vi "AddOrder.vi"(11 "buffer.in":u64[](array[numeric])=[2459274161843883858, 5279397646710161952, 5620492615227034656, 281474976710656, 0, 0, 0, 0, 0] format="%.0x") -> (3 "OrderBook.Command":T1={"type"=enum."AddOrder", "side"=66, "orderId "=3544385890602799695, "quantity"=20000, "symbol"=138719281473, "price"=1, "executed.qty"=0, "canceled.qty"=0, "remaining.qty"=0, "seconds"=0, "nanoseconds"=447000, "Add"=FALSE, "Edit"=FALSE, "Remove"=FALSE} {"symbol" format="%.0x"})   [LabVIEW 2020]
uses:
  builds/fpganow.common/orderbook.command.ctl
  builds/fpganow.common/orderbook.command.type.ctl
  Market.Data.Common/fpga/fpganow.common.fpga.lvlib
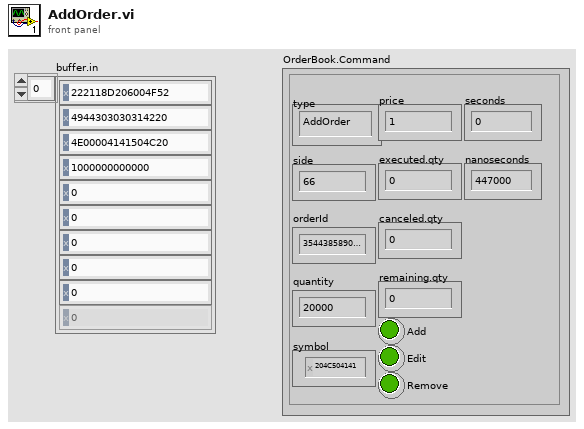
[diagram p1: front panel]
types:
  T1 = typedef "fpganow.common.fpga.lvlib/orderbook.command.ctl" = cluster{"type":T2, "side":u8, "orderId ":u64, "quantity":u32, "symbol":u64, "price":u64, "executed.qty":u32, "canceled.qty":u32, "remaining.qty":u32, "seconds":u64, "nanoseconds":u64, "Add":bool, "Edit":bool, "Remove":bool}
  T2 = typedef "fpganow.common.fpga.lvlib/orderbook.command.type.ctl" = enum8{"Time", "AddOrder", "OrderExecuted", "OrderExecutedAtPrice", "ReduceSize", "ModifyOrder", "DeleteOrder", "Get.Everything", "Get.All.Orders", "Get.Top"}
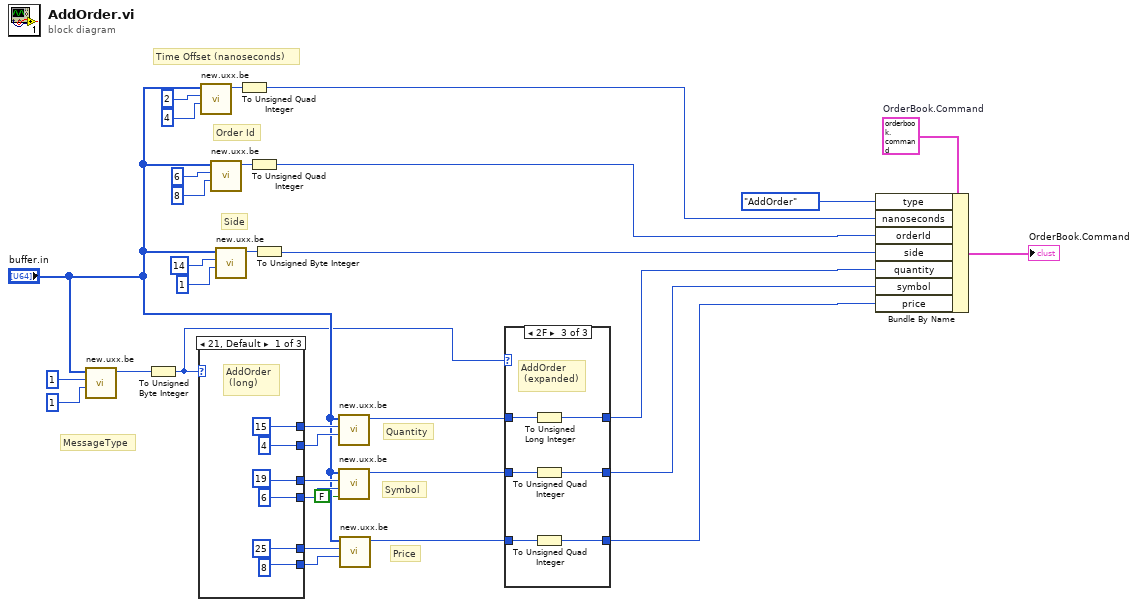
[diagram p0: block diagram]
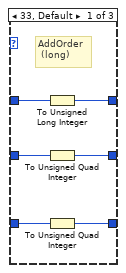
[diagram p2: hidden frame]
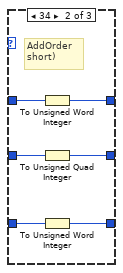
[diagram p3: hidden frame]
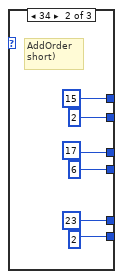
[diagram p4: hidden frame]
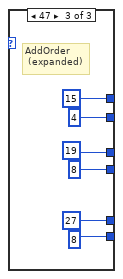
[diagram p5: hidden frame]
diagram:
  w30 = T1 {"type"=enum."AddOrder", "side"=0, "orderId "=0, "quantity"=0, "symbol"=0, "price"=0, "executed.qty"=0, "canceled.qty"=0, "remaining.qty"=0, "seconds"=0, "nanoseconds"=0, "Add"=FALSE, "Edit"=FALSE, "Remove"=FALSE}  # OrderBook.Command
  # "Price"
  # "Symbol"
  # "Quantity"
  # "Side"
  # "Order Id"
  # "Time Offset (nanoseconds)"
  # "MessageType"
  n1 = call "new.uxx.be.vi"("buffer (U64)"="buffer.in", "Start.Idx"=u8 1, "Length"=u8 1) -> ("Uxx.be"=w31:u64)  [unwired: 7 in]
  n2 = To Unsigned Byte Integer(number=w31) -> (unsigned 8bit integer=w5:u8)
  n3 = case shown="21, Default" w5 {
    tunnel: [u8 15 ("Start.Idx") u8 15 ("Start.Idx") u8 15 ("Start.Idx")] -> w12
    tunnel: [u8 4 ("Length") u8 2 ("Length") u8 4 ("Length")] -> w11
    tunnel: [u8 19 ("Start.Idx") u8 17 ("Start.Idx") u8 19 ("Start.Idx")] -> w10
    tunnel: [u8 6 ("Length") u8 6 ("Length") u8 8 ("Length")] -> w9
    tunnel: [u8 25 ("Start.Idx") u8 23 ("Start.Idx") u8 27 ("Start.Idx")] -> w8
    tunnel: [u8 8 ("Length") u8 2 ("Length") u8 8 ("Length")] -> w7
    frame 33, Default {
      # "AddOrder\n (long)"
    }
    frame 34 {
      # "AddOrder \nshort)"
    }
    frame 47 {
      # "AddOrder\n (expanded)"
    }
  }
  n4 = call "new.uxx.be.vi"("buffer (U64)"="buffer.in", "Start.Idx"=u8 2, "Length"=u8 4) -> ("Uxx.be"=w25:u64)  [unwired: 7 in]
  n5 = call "new.uxx.be.vi"("buffer (U64)"="buffer.in", "Start.Idx"=u8 6, "Length"=u8 8) -> ("Uxx.be"=w22:u64)  [unwired: 7 in]
  n6 = call "new.uxx.be.vi"("buffer (U64)"="buffer.in", "Start.Idx"=u8 14, "Length"=u8 1) -> ("Uxx.be"=w19:u64)  [unwired: 7 in]
  n7 = To Unsigned Quad Integer(1:w25) -> (0:w15:u64)
  n8 = To Unsigned Quad Integer(1:w22) -> (0:w14:u64)
  n9 = To Unsigned Byte Integer(number=w19) -> (unsigned 8bit integer=w13:u8)
  n10 = call "new.uxx.be.vi"("buffer (U64)"="buffer.in", "Start.Idx"=w12, "Length"=w11) -> ("Uxx.be"=w18:u64)  [unwired: 7 in]
  n11 = call "new.uxx.be.vi"("buffer (U64)"="buffer.in", "Start.Idx"=w10, "Length"=w9, "Big.Endian?"=FALSE) -> ("Uxx.be"=w17:u64)  [unwired: 6 in]
  n12 = call "new.uxx.be.vi"("buffer (U64)"="buffer.in", "Start.Idx"=w8, "Length"=w7) -> ("Uxx.be"=w16:u64)  [unwired: 7 in]
  n13 = case shown="2F" w5 {
    tunnel: [w54 w60 w66] -> w4
    tunnel: [w53 w59 w65] -> w3
    tunnel: [w52 w58 w64] -> w2
    tunnel: w18 -> [w57 w61 w68]
    tunnel: w16 -> [w55 w63 w69]
    tunnel: w17 -> [w56 w62 w67]
    frame 33, Default {
      # "AddOrder\n (long)"
      n14 = To Unsigned Long Integer(number=w57) -> (unsigned 32bit integer=w54:u32)
      n15 = To Unsigned Quad Integer(1:w56) -> (0:w53:u64)
      n16 = To Unsigned Quad Integer(1:w55) -> (0:w52:u64)
    }
    frame 34 {
      # "AddOrder \nshort)"
      n17 = To Unsigned Word Integer(number=w61) -> (unsigned 16bit integer=w60:u16)
      n18 = To Unsigned Quad Integer(1:w62) -> (0:w59:u64)
      n19 = To Unsigned Word Integer(number=w63) -> (unsigned 16bit integer=w58:u16)
    }
    frame 47 {
      # "AddOrder\n (expanded)"
      n20 = To Unsigned Long Integer(number=w68) -> (unsigned 32bit integer=w66:u32)
      n21 = To Unsigned Quad Integer(1:w67) -> (0:w65:u64)
      n22 = To Unsigned Quad Integer(1:w69) -> (0:w64:u64)
    }
  }
  n23 = Bundle By Name(cluster=w30, "type"=orderbook.command.type."AddOrder" ("OrderBook Command"), "nanoseconds"=w15, "orderId"=w14, "side"=w13, "quantity"=w4, "symbol"=w3, "price"=w2) -> (→"OrderBook.Command":T1)
